vi "Get String.vi"(8 "error in (no error)":errorcluster, 9 "Data Type (default value)":string, 10 "Offset":i32, 11 "JSON":string) -> (0 "error out":errorcluster, 1 "String":string, 2 "Offset past match":i32)   [LabVIEW 2017, in "JSONtext.lvlib"]
uses:
  JSONtext.lvlib
  Unescape JSON string.vi
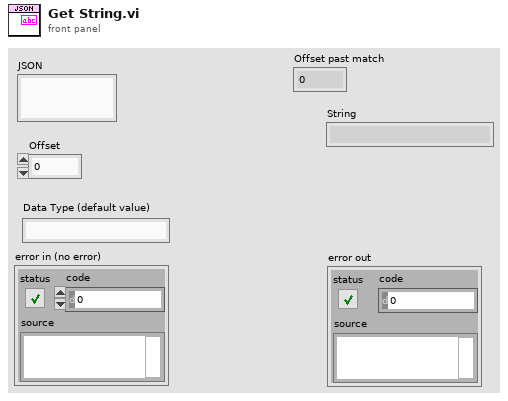
[diagram p1: front panel]
types:
  T1 = typedef "JSONtext.lvlib/Parsing State.ctl" = enum16{"Parser Error", "Object", "Array", "String", "Number/Other", "Leading Whitespace", "Object end", "Array end", "Value end"}
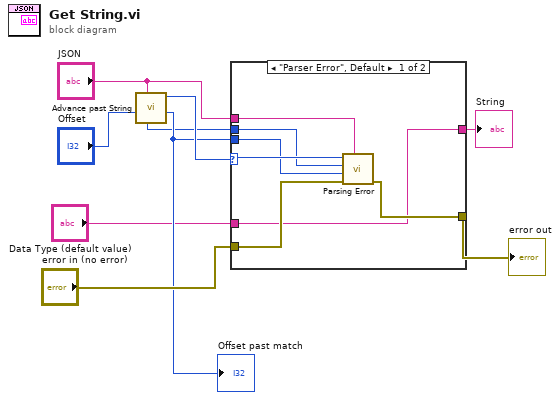
[diagram p0: block diagram]
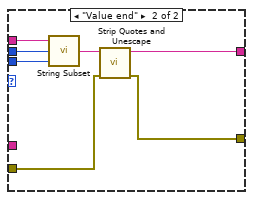
[diagram p2: hidden frame]
diagram:
  n1 = call "Advance past String.vi"("JSON"="JSON", "Offset"="Offset") -> ("Offset past match"=w3:i32, "State"=w7:T1, "Value start out"=w2:i32)  [unwired: 7 in]
  "Offset past match" <- w3
  n2 = case shown="\"Parser Error\", Default" w7 {
    selector: w7 -> [w14 _]
    tunnel: "JSON" -> [w11 w22]
    tunnel: [w16 w20] -> w6
    tunnel: "error in (no error)" -> [w15 w21]
    tunnel: [w10 w19] -> w4
    tunnel: w2 -> [w13 w18]
    tunnel: w3 -> [w12 w17]
    tunnel: "Data Type (default value)" -> [w10 _]
    frame "Parser Error", Default {
      n3 = call "Parsing Error.vi"("JSON"=w11, "error in (no error)"=w15, "Offset past match"=w12, "Value start"=w13, "State"=w14) -> ("error out"=w16:errorcluster)  [unwired: 6 in]
    }
    frame "Value end" {
      n4 = call "String Subset.vi"("Offset past End"=w17, "Start offset"=w18, "JSON"=w22) -> ("substring"=w23:string)  [unwired: 2 in]
      n5 = call "Strip Quotes and Unescape.vi"("error in (no error)"=w21, "String"=w23) -> ("error out"=w20:errorcluster, "result string"=w19:string)  [unwired: 8 in]
    }
  }
  "error out" <- w6
  "String" <- w4
